vi "Get DNRPs.vi"(8 "error in (no error)":errorcluster, 11 "DNR rack resource":string) -> (0 "error out":errorcluster {"code" format="%x"}, 3 "DNRPs":i32[](array[numeric]))   [LabVIEW 8.6]
uses:
  vi.lib/UeiDaq/UeiDaqCreateEnumSession.vi
  <libdir>/resource/objmgr/ueidaq.rc
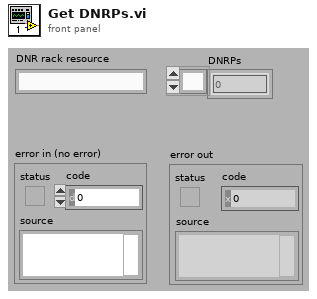
[diagram p1: front panel]
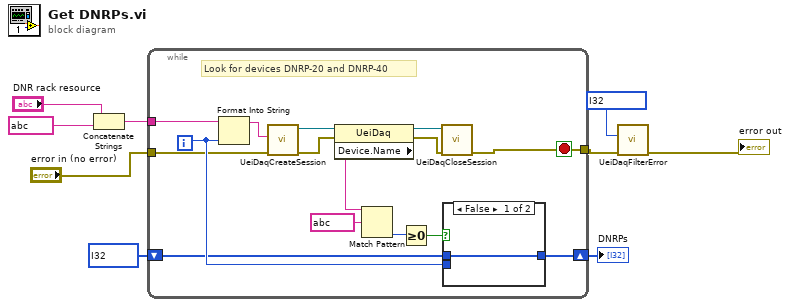
[diagram p0: block diagram]
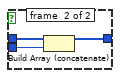
[diagram p2: hidden frame]
diagram:
  n1 = Concatenate Strings("DNR rack resource", string ? ("string")) -> (w7:string)
  n2 = while {
    tunnel: w7 -> [w21]
    shift-right: [w13] -> w5
    shift-left: i32[] ? -> [w12]
    tunnel: [w11] -> w4
    tunnel: "error in (no error)" -> [w10]
    i -> [w14]
    stop <- w11 stop-if-true
    # "Look for devices DNRP-20 and DNRP-40"
    n3 = Format Into String(format string=w21, w14) -> (resulting string=w22:string)  [unwired: 2 in, 1 out]
    n4 = call-poly "UeiDaqCreateSession.vi"("error in (no error)"=w10, "Resource"=w22) -> ("error out"=w23:errorcluster, "UeiDaq Refnum Out"=w24:refnum<k20>)  [unwired: 1 in, 7 out]
    n5 = property class="UeiDaq"(reference=w24, error in=w23) -> (reference out=w20:refnum<k20>, error out=w19:errorcluster, "Device.Name"=w17:string)
    n6 = Match Pattern(string=w17, regular expression=string ?) -> (offset past match=w16:i32)  [unwired: 4 out]
    n7 = Greater Or Equal To 0?(x=w16) -> (x >= 0?=w15:bool)
    n8 = call "UeiDaqCloseSession.vi"("error in (no error)"=w19, "UeiDaq Refnum In"=w20) -> ("error out"=w11:errorcluster)  [unwired: 9 out]
    n9 = case shown="False" w15 {
      tunnel: w14 -> [_ w28]
      tunnel: [w25 w27] -> w13
      tunnel: w12 -> [w25 w26]
      frame #0 {
      }
      frame #1 {
        n10 = Build Array (concatenate)(w26, w28) -> (w27:i32[])
      }
    }
  }
  "DNRPs" <- w5
  n11 = call "UeiDaqFilterError.vi"("error in (no error)"=w4, "Error to filter"=i32 ?) -> ("error out"=→"error out":errorcluster)  [unwired: 1 in, 8 out]
